vi "sc5511a_store_default_state.vi"(0 "deviceHandle":u32 format="%.0x", 5 "error in":errorcluster) -> (14 "deviceHandle":u32 format="%.0x", 19 "error out":errorcluster)   [LabVIEW 2010]
uses:
  sc5511a_rs232.dll
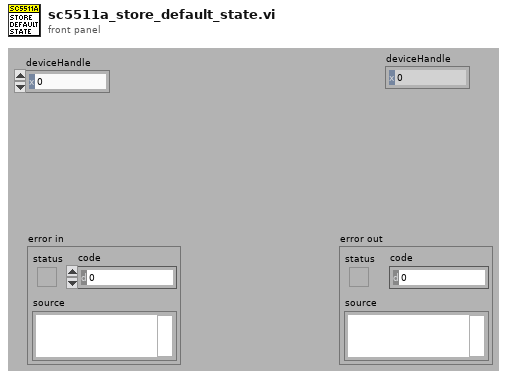
[diagram p1: front panel]
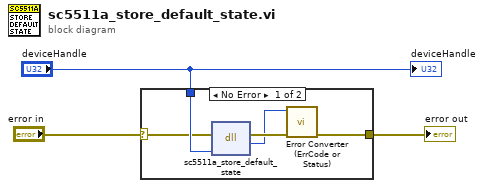
[diagram p0: block diagram]
diagram:
  n1 = case shown="No Error" "error in" {
    selector: "error in" -> [w4 w9]
    tunnel: [w8 w9] -> w3
    tunnel: "deviceHandle" -> [w5 _]
    frame No Error {
      n2 = dll-call lib="sc5511a_rs232.dll" fn="sc5511a_store_default_state"(error in=w4, "deviceHandle"=w5) -> (error out=w7:errorcluster, "return type"=w6:i32)  [unwired: 3 in, 1 out]
      n3 = call "Error Converter (ErrCode or Status).vi"("error in (no error)"=w7, "error code"=w6) -> ("error out"=w8:errorcluster)  [unwired: 9 in]
    }
    frame Error {
    }
  }
  "error out" <- w3
  "deviceHandle" <- "deviceHandle"
